vi "Proyecto finall.vi"() -> ()   [LabVIEW 2023]
uses:
  <vilib>/userDefined/High Color/IMAQdx.ctl
  <vilib>/DAQmx/write.llb/DAQmx Write (Digital 1D Bool NChan 1Samp 1Line).vi
  <vilib>/addons/database/Connection.llb/DB Tools Open Connec (Path).vi
  <vilib>/addons/database/Connection.llb/Conn Execute.vi
  <vilib>/addons/database/Recordset.llb/Rec Fetch Recordset Data (R).vi
  <vilib>/addons/database/Recordset.llb/Rec Destroy - Connection.vi
  <vilib>/DAQmx/miscellaneous.llb/DAQmx Fill In Error Info.vi
  <vilib>/addons/database/NI_Database_API.lvlib
  <vilib>/vision/driver/NI_Vision_Acquisition_Software.lvlib
panel:
  out "crujos 2":u16(ring)=1
  out "doros 2":u16(ring)=1
  out "cheetines 2":u16(ring)=1
  out "Gansito 2":u16(ring)=1
  out "Chips 2":u16(ring)=1
  out "Takis 2":u16(ring)=1
  out "SALDO":i32
  in  "Stop Button":bool
  out "Total Carrito":dbl=19.0
  in  "crujitos1":dbl min=0.0
  in  "doritos1":dbl min=0.0
  in  "chettos1":dbl min=0.0
  in  "chips1":dbl min=0.0
  in  "gansito1":dbl min=0.0
  in  "takis1":dbl min=0.0
  in  "STOP PROGRAMA":bool
  out "Takis":u16(ring)=1
  in  "disponibilidad tak":dbl=3.0 min=0.0 max=3.0
  in  "SaldoAux":dbl=100.0
  in  "Comprar":bool
  out "crujos":u16(ring)=3
  in  "disponibilidad cruji":dbl=3.0 min=0.0 max=3.0
  in  "crujitos":bool
  out "doros":u16(ring)=2
  in  "disponibilidad dori":dbl=3.0 min=0.0 max=3.0
  in  "doritos":bool
  out "cheetines":u16(ring)=2
  in  "disponibilidad chee":dbl=3.0 min=0.0 max=3.0
  in  "cheetos":bool
  out "String (OCR/OCV 1)":string="      "
  in  "File Path (OCR/OCV 1)":path=path "C:/Users/miagu/OneDrive/Escritorio/NUMBER.abc"
  out "Image":T1(plugin-control)
  out "Gansito":u16(ring)=2
  out "Chips":u16(ring)=2
  in  "disponibilidad gans":dbl=3.0 min=0.0 max=3.0
  in  "Disponibilidad chi":dbl=3.0 min=0.0 max=3.0
  in  "UDL":path=path "C:/Users/Dell/Desktop/maquina.udl"
  in  "gansito":bool
  in  "chips":bool
  in  "takis":bool
  out "Numeric 3":i32
  # "Carrito"
  # "Agregar Objetos"
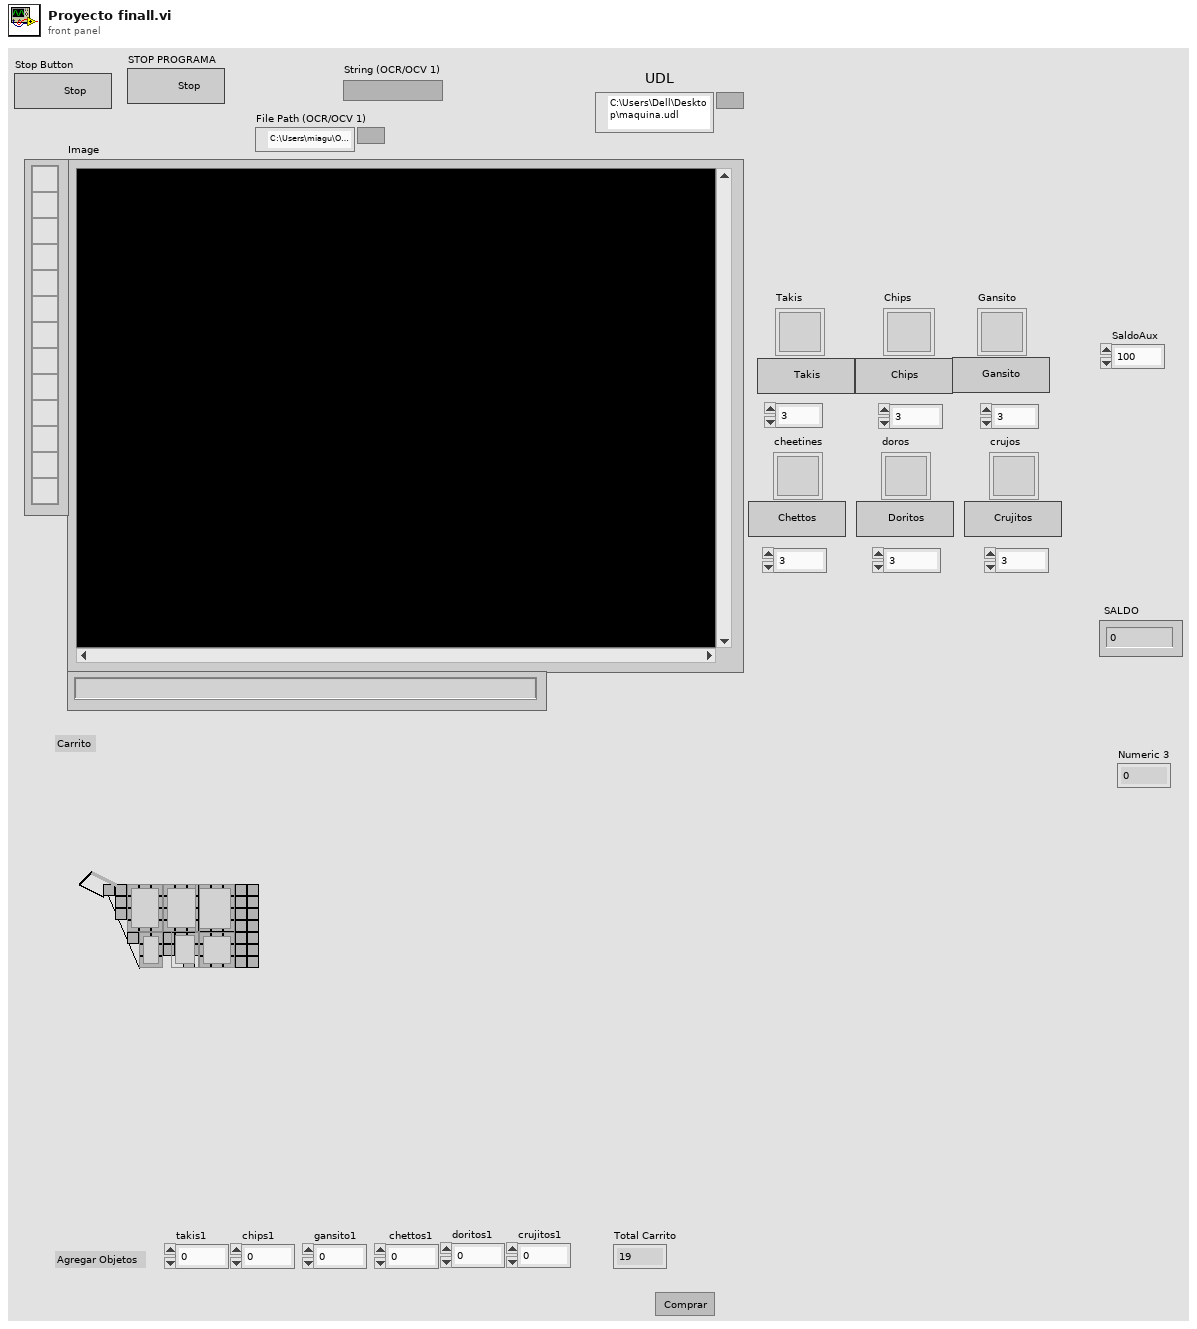
[diagram p1: front panel]
types:
  T1 = typedef "IMAQ Image.ctl" = refnum<image>
  T2 = cluster{"Threshold Data":cluster{"Method":enum16{"Fixed Range", "Uniform", "Linear", "Non Linear", "Local", "Color"}, "Looking for":u32, "Color Mode":u32, "Kernel Size":cluster{"Width":i32, "Height":i32}, "Ranges":cluster{"Min":i32, "Max":i32}[]}, "Reject Border":bool, "Number Of Erosions":i32, "Size & Spacing":cluster{"Segment Algorithm":u16, "Min Bounding Rect Width":i32, "Max Bounding Rect Width":i32, "Min Bounding Rect Height":i32, "Max Bounding Rect Height":i32, "Min Character Size":i32, "Max Character Size":i32, "Min Char Spacing":i32, "Max Horiz Element Spacing":i32, "Max Vert Element Spacing":i32, "Max Space Distance":i32}, "Read Options":cluster{"Read Strategy":i32, "Read Resolution":i32, "Scale Dependant":bool, "Aspect Ratio":i32, "Acceptance Level":i32, "Substitution Character":string, "MultiLine":bool}, "Valid Characters":cluster{"Pre-defined characters":i32, "User-defined characters":string}[], "Use Text Pattern":bool, "Orientation":u32, "# Lines Expected":u32, "Number of Blocks":i32}
  T3 = typedef "IMAQdx.ctl" = refnum<k21>
  T4 = cluster{"Global Rectangle":i32[], "Contours":cluster{"Contour Type":u32, "ROI Type":u32, "Points":i32[]}[]}
  T5 = typedef "NI_Database_API.lvlib/Conn ObjectReference.ctl" = refnum<k1>
  T6 = typedef "NI_Database_API.lvlib/Rec ObjectReference.ctl" = refnum<k1>
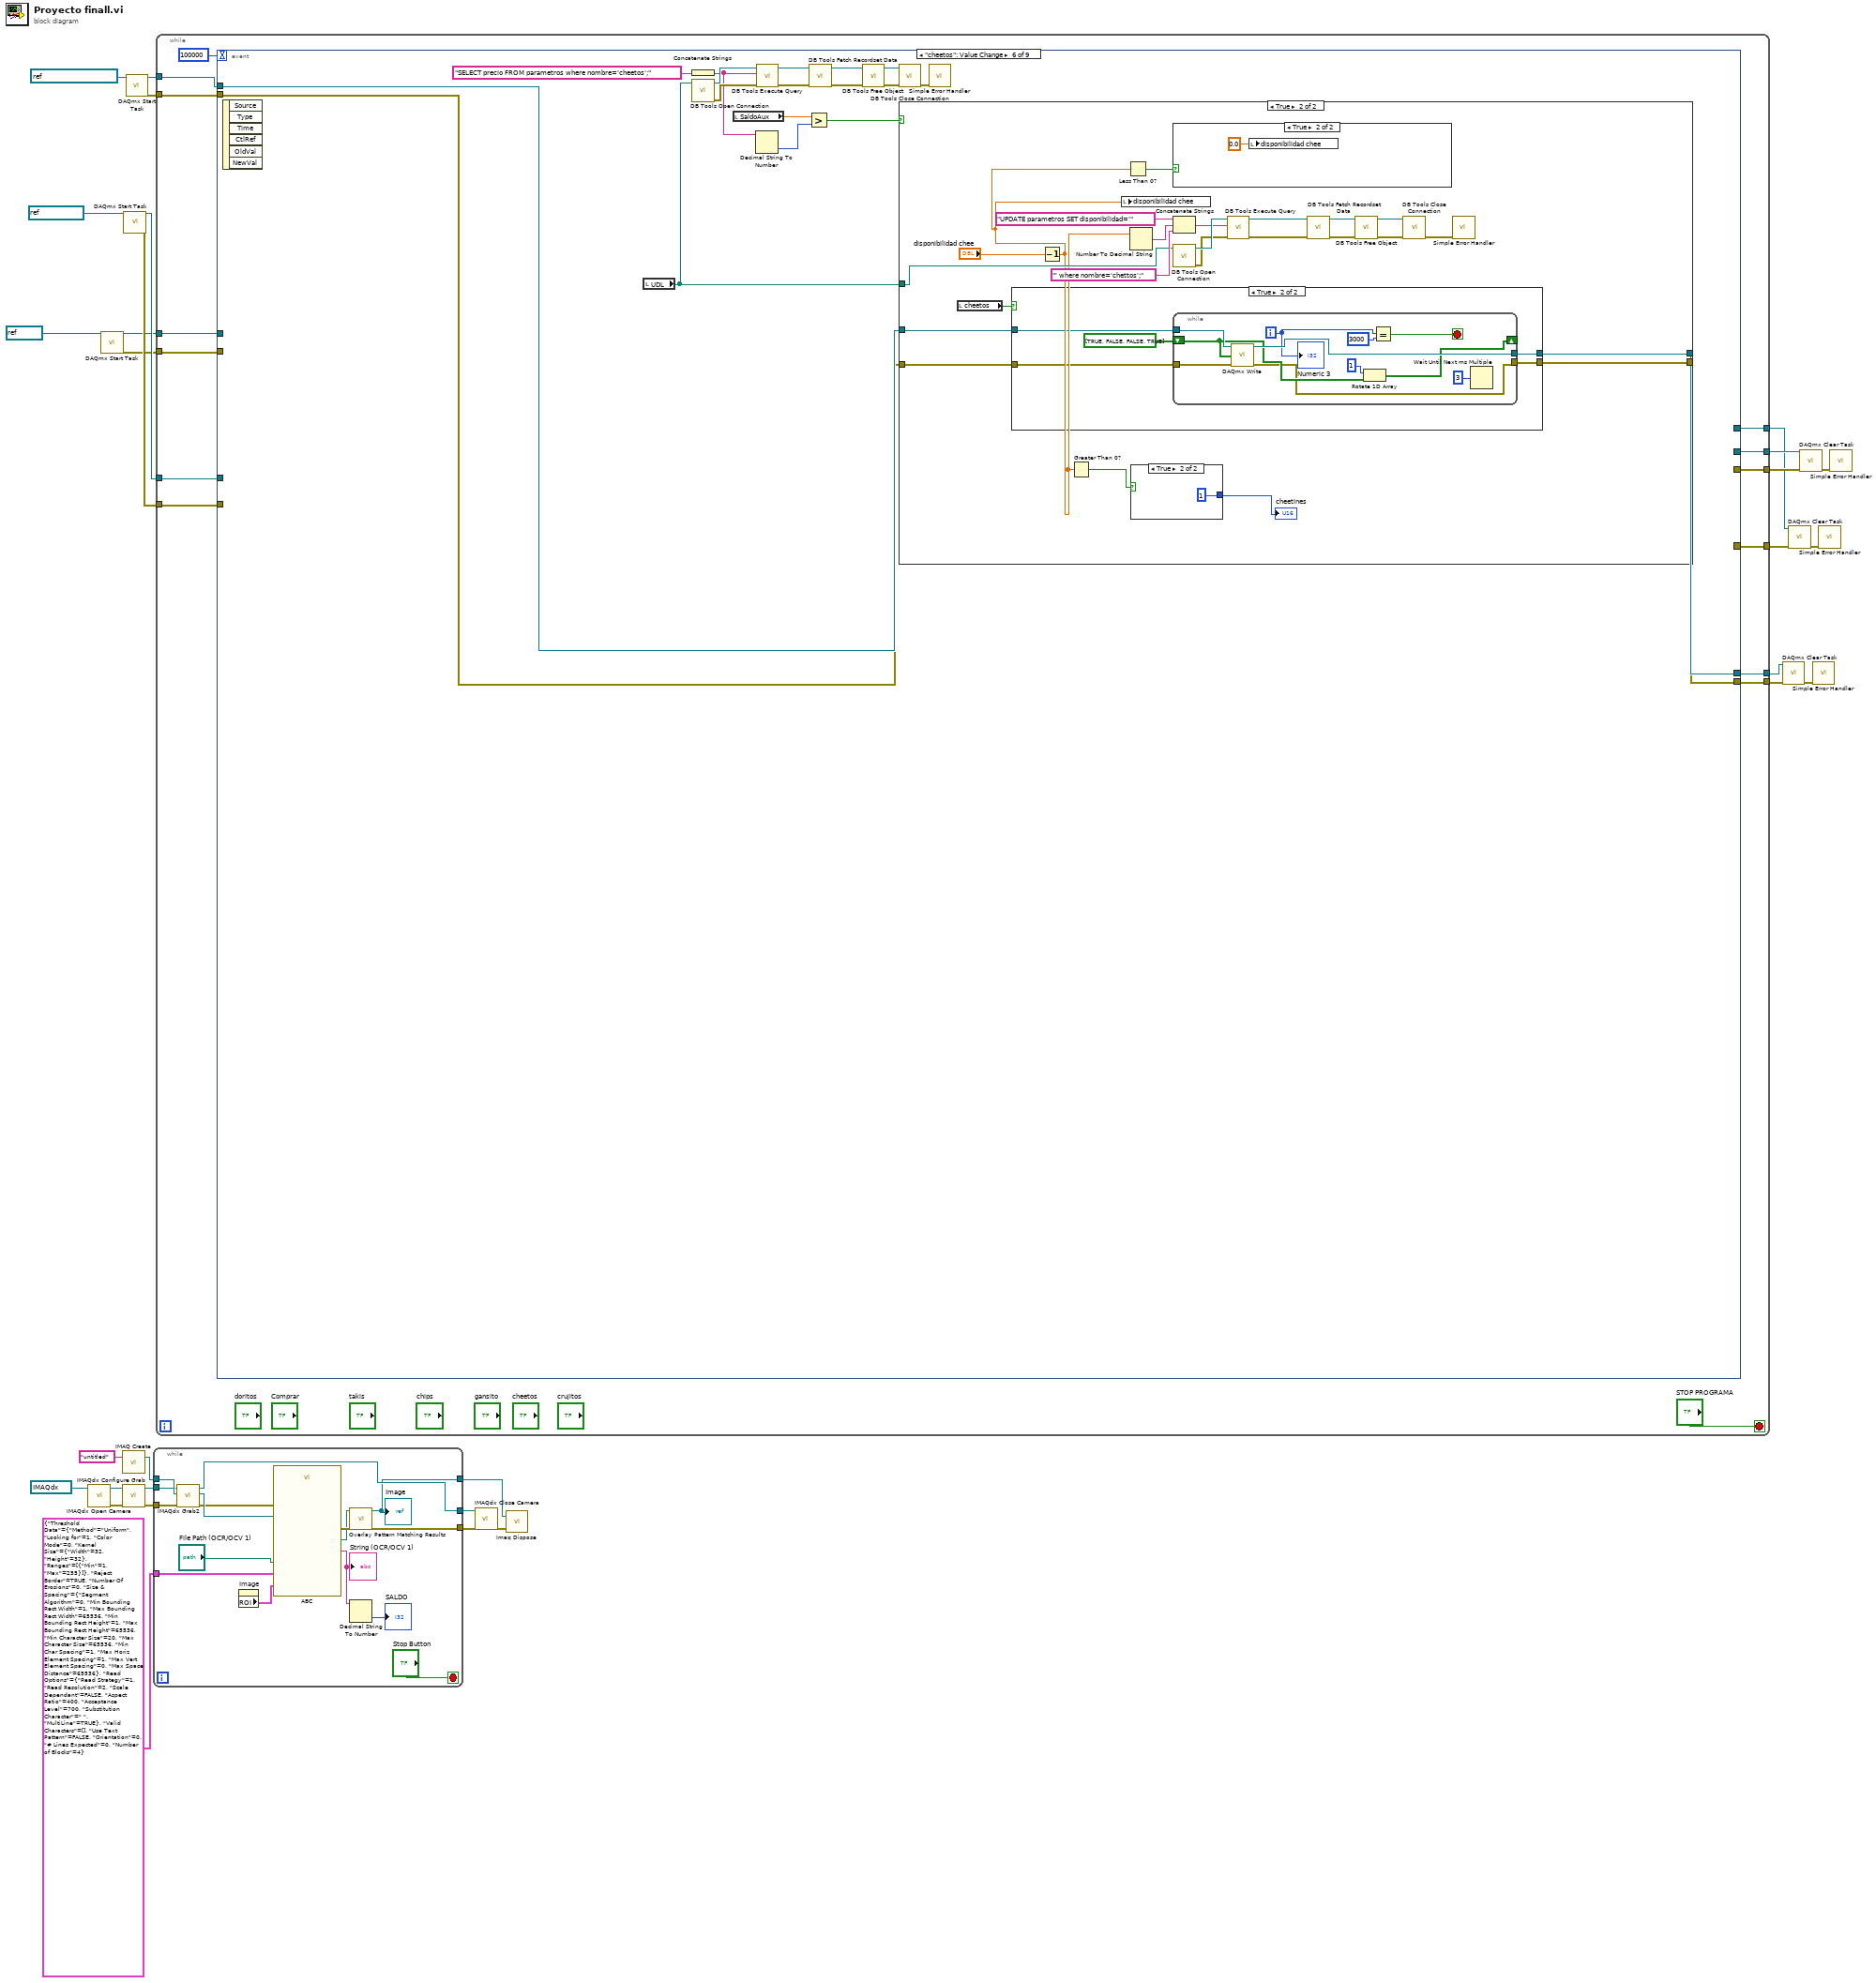
[diagram p0: block diagram]
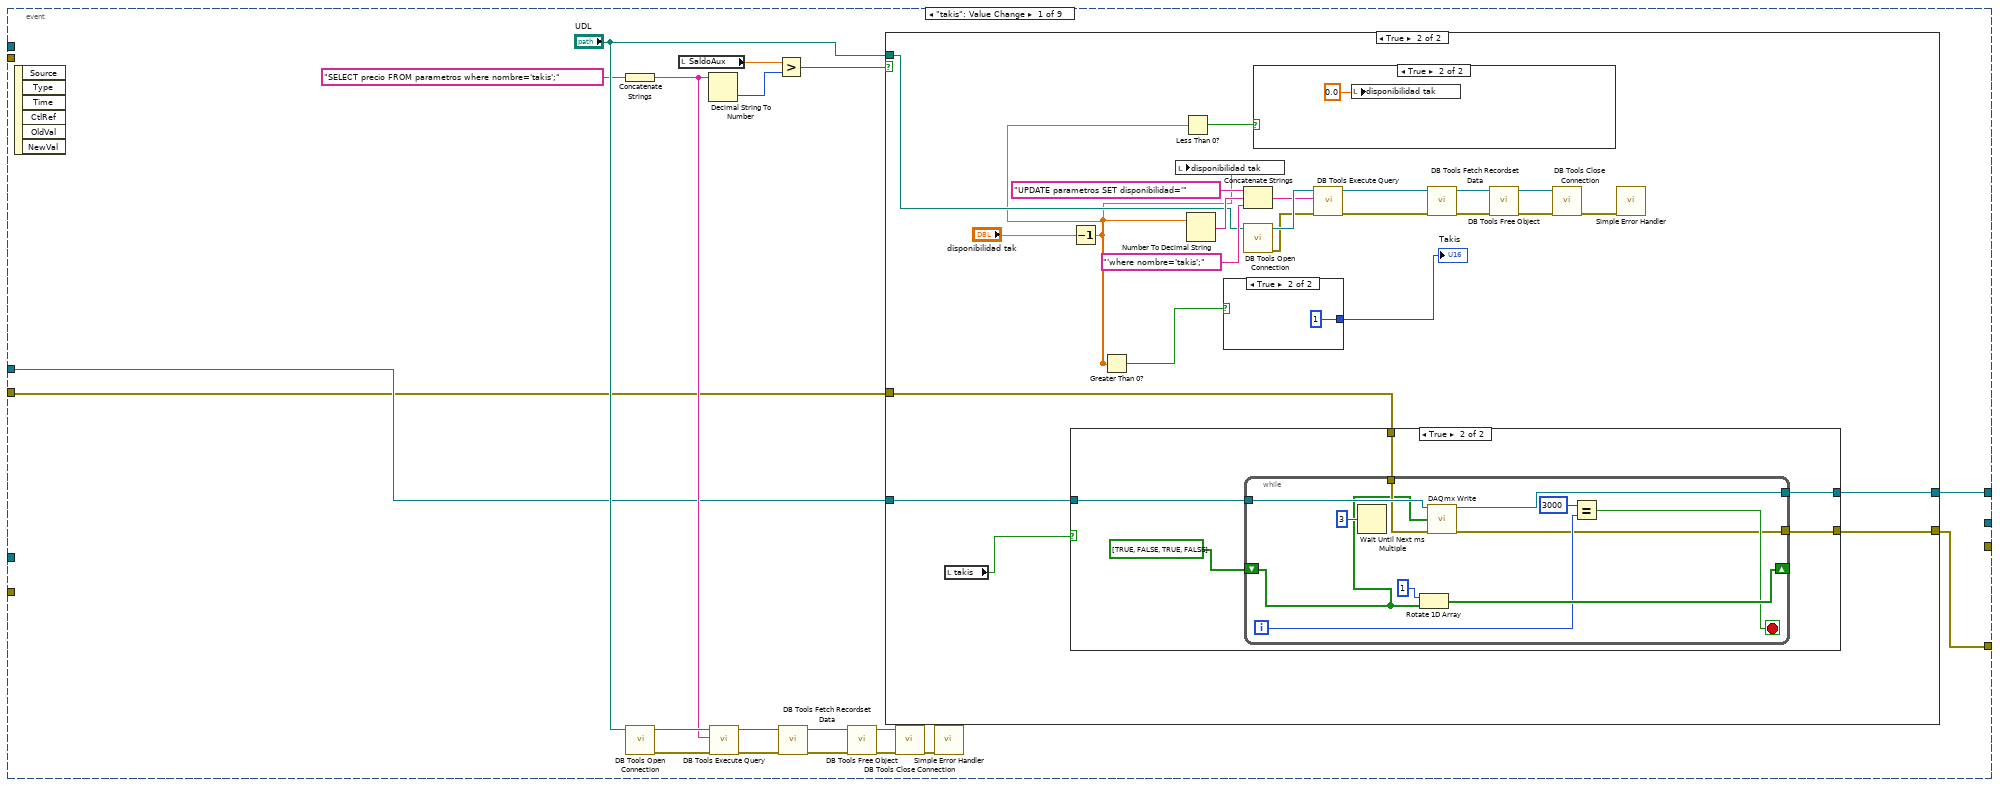
[diagram p2: hidden frame]
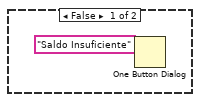
[diagram p3: hidden frame]
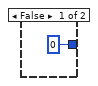
[diagram p5: hidden frame]
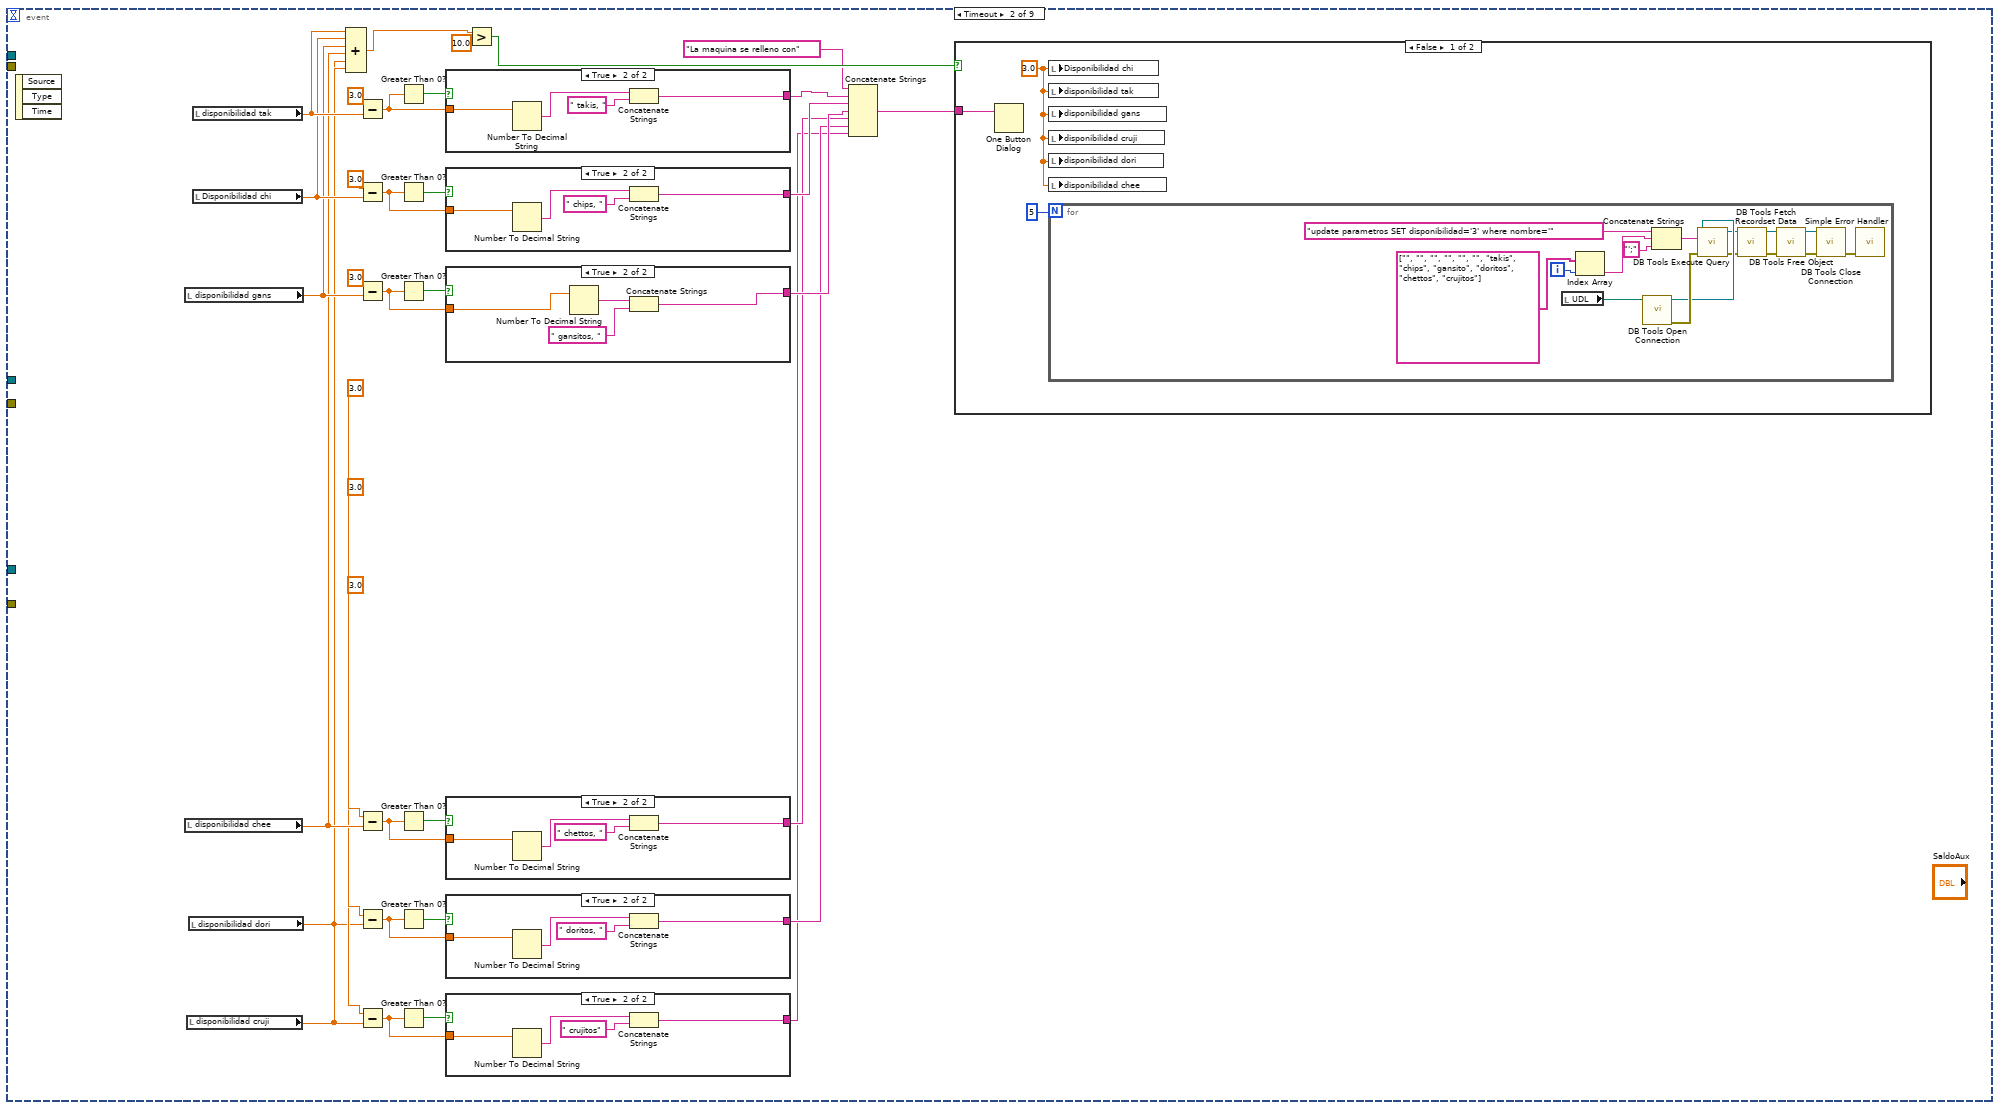
[diagram p7: hidden frame]
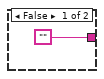
[diagram p8: hidden frame]
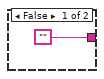
[diagram p9: hidden frame]
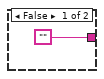
[diagram p10: hidden frame]
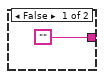
[diagram p11: hidden frame]
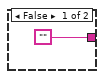
[diagram p12: hidden frame]
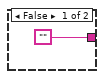
[diagram p13: hidden frame]
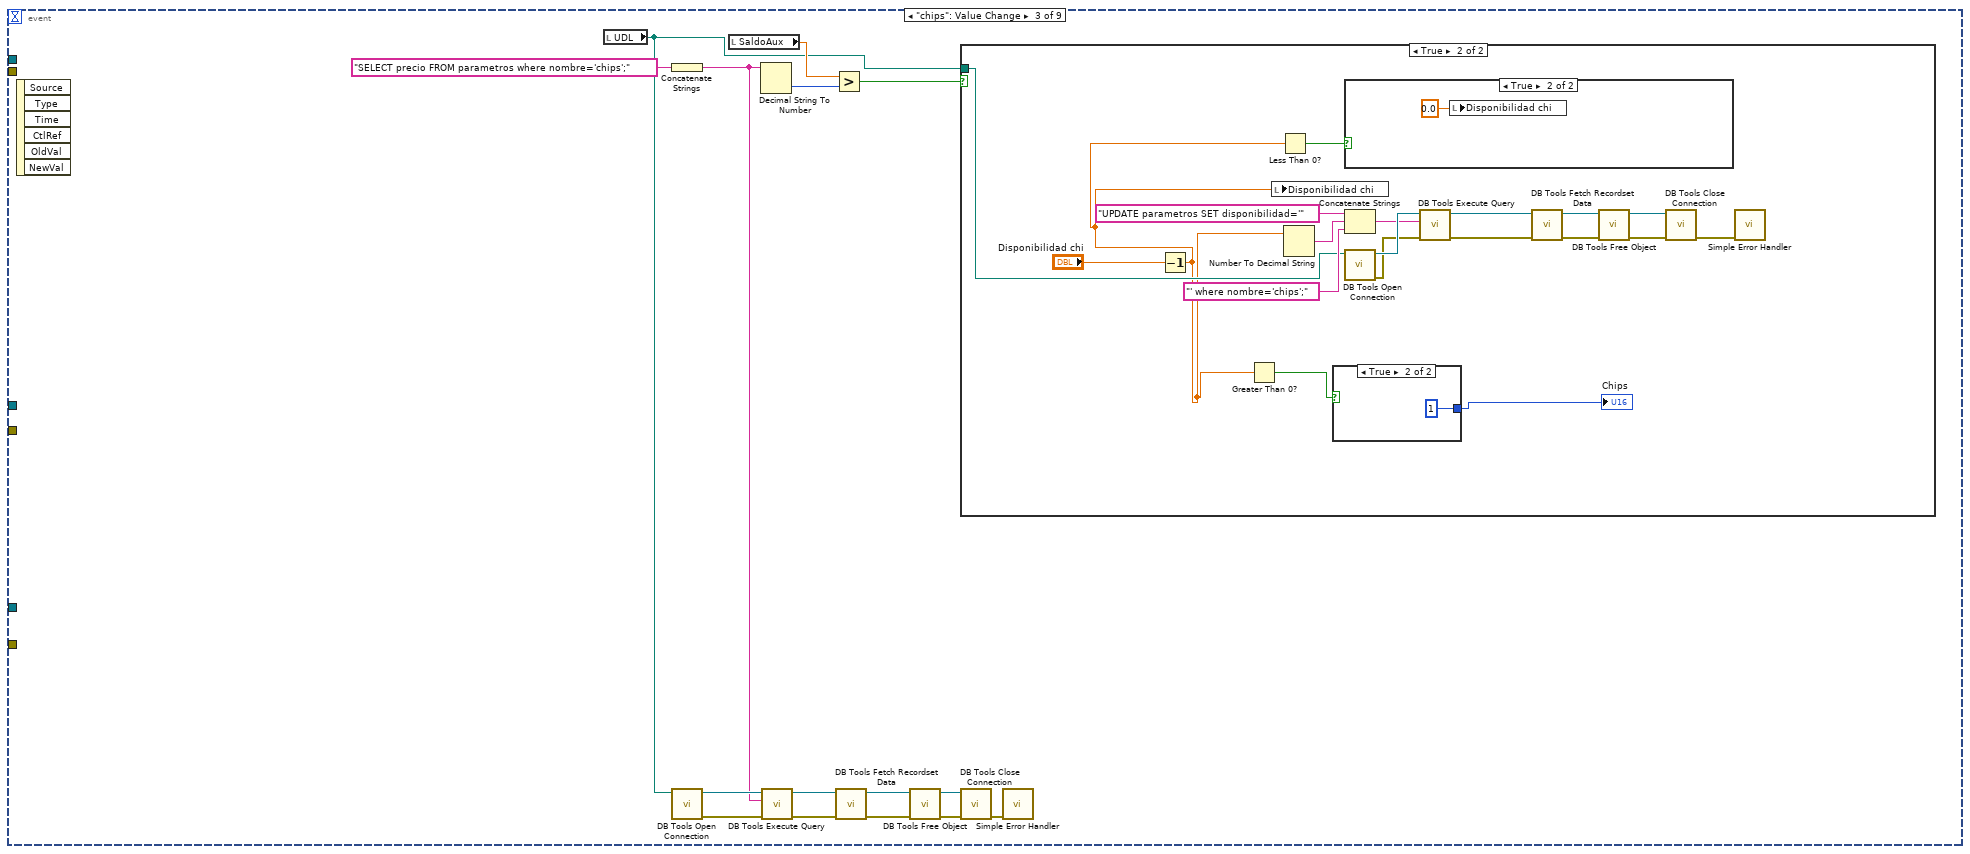
[diagram p15: hidden frame]
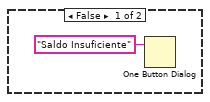
[diagram p16: hidden frame]
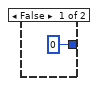
[diagram p17: hidden frame]
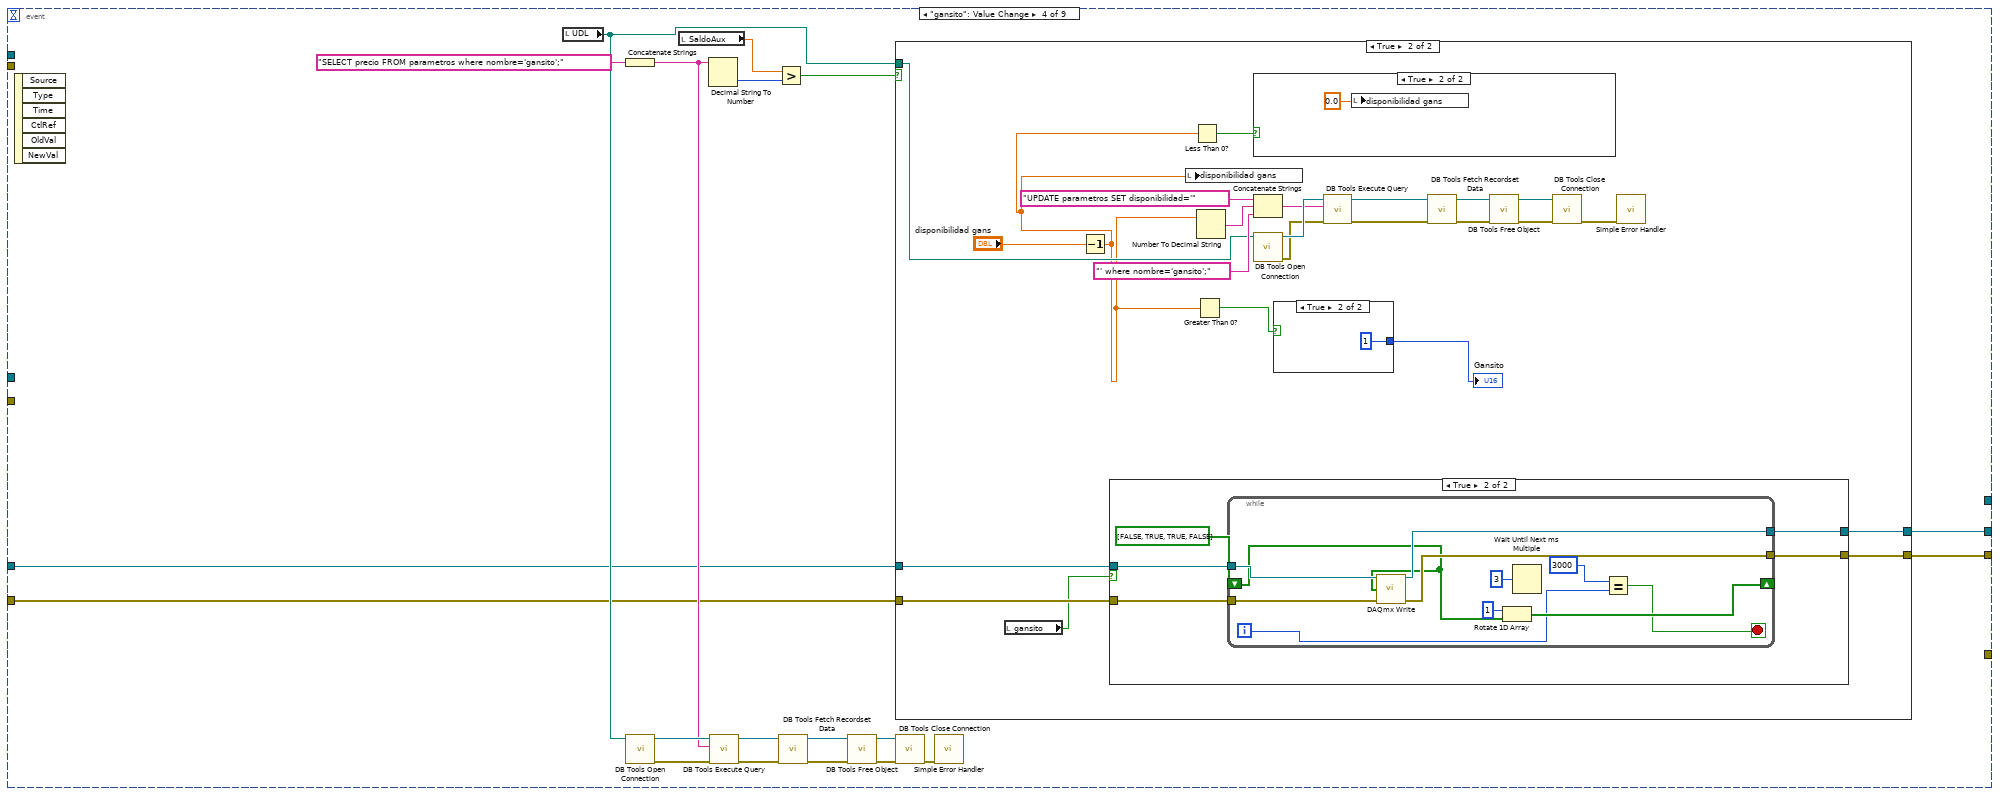
[diagram p19: hidden frame]
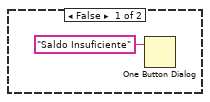
[diagram p20: hidden frame]
diagram:
  n1 = call <vilib>:"IMAQdx Open Camera.vi"("Session In"=T3 "cam1") -> ("error out"=w28:errorcluster, "Session Out"=w29:T3)  [unwired: 9 in]
  n2 = call <vilib>:"DAQmx Start Task.vi"("task/channels in"=refnum<k21> "out3") -> ("task out"=w5:refnum<k21>, "error out"=w4:errorcluster)  [unwired: 13 in]
  n3 = call "IMAQ Create"("Image Name"="untitled") -> ("New Image"=w18:T1)  [unwired: 4 in, 1 out]
  n4 = call <vilib>:"IMAQdx Configure Grab.vi"("error in"=w28, "Session In"=w29) -> ("error out"=w19:errorcluster, "Session Out"=w17:T3)  [unwired: 8 in]
  n5 = call <vilib>:"DAQmx Start Task.vi"("task/channels in"=refnum<k21> "OutTask2") -> ("task out"=w8:refnum<k21>, "error out"=w7:errorcluster)  [unwired: 13 in]
  n6 = call <vilib>:"DAQmx Start Task.vi"("task/channels in"=refnum<k21> "MyDigitalOutTask") -> ("task out"=w21:refnum<k21>, "error out"=w20:errorcluster)  [unwired: 13 in]
  n7 = while {
    tunnel: w19 -> [w45]
    tunnel: w18 -> [w44]
    tunnel: w17 -> [w43]
    tunnel: [w42] -> w16
    tunnel: T2 {"Threshold Data"={"Method"=enum."Uniform", "Looking for"=1, "Color Mode"=0, "Kernel Size"={"Width"=32, "Height"=32}, "Ranges"=[{"Min"=1, "Max"=255}]}, "Reject Border"=TRUE, "Number Of Erosions"=0, "Size & Spacing"={"Segment Algorithm"=0, "Min Bounding Rect Width"=1, "Max Bounding Rect Width"=65536, "Min Bounding Rect Height"=1, "Max Bounding Rect Height"=65536, "Min Character Size"=20, "Max Character Size"=65536, "Min Char Spacing"=1, "Max Horiz Element Spacing"=1, "Max Vert Element Spacing"=0, "Max Space Distance"=65536}, "Read Options"={"Read Strategy"=1, "Read Resolution"=2, "Scale Dependant"=FALSE, "Aspect Ratio"=400, "Acceptance Level"=700, "Substitution Character"=" ", "MultiLine"=TRUE}, "Valid Characters"=[], "Use Text Pattern"=FALSE, "Orientation"=0, "# Lines Expected"=0, "Number of Blocks"=4} ("Parameters (OCR/OCV 1)") -> [w38]
    tunnel: [w32] -> w14
    tunnel: [w31] -> w13
    stop <- "Stop Button" stop-if-true
    n8 = call <vilib>:"IMAQdx Grab2.vi"("error in"=w45, "Image In"=w44, "Session In"=w43) -> ("error out"=w37:errorcluster, "Image Out"=w41:T1, "Session Out"=w42:T3)  [unwired: 5 in, 1 out]
    n9 = property on="Image" class="ImageControl"() -> ("ROI"=w40:T4)  [unwired: 2 in, 2 out]
    n10 = call "ABC.vi"("Image In"=w41, "ROI Descriptor (OCR/OCV 1)"=w40, "File Path (OCR/OCV 1)"="File Path (OCR/OCV 1)", "Parameters (OCR/OCV 1)"=w38, "error in"=w37) -> ("Image Out"=w33:T1, "String (OCR/OCV 1)"=w35:string, "error out"=w34:errorcluster)  [unwired: 20 in]
    "String (OCR/OCV 1)" <- w35
    n11 = call "Overlay Pattern Matching Results.vi"("error in"=w34, "Image"=w33) -> ("error out"=w32:errorcluster, "Image Out"=w31:T1)  [unwired: 8 in]
    "Image" <- w31
    n12 = Decimal String To Number(string=w35) -> (number=→"SALDO":i32)  [unwired: 2 in, 1 out]
  }
  n13 = while {
    tunnel: [w59] -> w24
    tunnel: [w58] -> w23
    tunnel: w21 -> [w57]
    tunnel: w20 -> [w56]
    tunnel: [w54] -> w11
    tunnel: [w53] -> w9
    tunnel: w8 -> [w52]
    tunnel: w7 -> [w51]
    tunnel: w5 -> [w50]
    tunnel: w4 -> [w49]
    tunnel: [w48] -> w2
    tunnel: [w47] -> w1
    stop <- "STOP PROGRAMA" stop-if-true
    n14 = event shown="[5] \"cheetos\": Value Change" {
      selector: _ -> [_ _ _ _ _ _ _ _ _]
      dyn-events: _ -> [_ _ _ _ _ _ _ _ _]
      timeout: 100000 -> [_ _ _ _ _ _ _ _ _]
      tunnel: [_ _ _ _ _ w459 _ _ _] -> w59
      tunnel: [_ _ _ _ _ w458 _ _ _] -> w58
      tunnel: w57 -> [_ _ _ _ _ w457 _ _ _]
      tunnel: w56 -> [_ _ _ _ _ w456 _ _ _]
      tunnel: [_ _ _ w249 _ _ _ _ _] -> w54
      tunnel: [_ _ _ w248 _ _ _ _ _] -> w53
      tunnel: w52 -> [_ _ _ w247 _ _ _ _ _]
      tunnel: w51 -> [_ _ _ w246 _ _ _ _ _]
      tunnel: w50 -> [w64 _ _ _ _ _ _ _ _]
      tunnel: w49 -> [w63 _ _ _ _ _ _ _ _]
      tunnel: [w62 _ _ _ _ _ _ _ _] -> w48
      tunnel: [w61 _ _ _ _ _ _ _ _] -> w47
      event "takis": Value Change {
        n15 = event-data() -> ()  [unwired: 1 in, 6 out]
        n16 = Concatenate Strings("SELECT precio FROM parametros where nombre='takis';") -> (w65:string)
        n17 = call-poly <vilib>:"DB Tools Open Connection.vi"("connection information"="UDL") -> ("error out"=w75:errorcluster, "connection reference"=w74:T5)  [unwired: 7 in]
        n18 = local read "SaldoAux"() -> (w69:dbl)
        n19 = Decimal String To Number(string=w65) -> (number=w70:i32)  [unwired: 2 in, 1 out]
        n20 = call-poly <vilib>:"DB Tools Execute Query.vi"("error in (no error)"=w75, "SQL query"=w65, "connection reference"=w74) -> ("error out"=w79:errorcluster, "recordset reference"=w73:T6)  [unwired: 5 in]
        n21 = Greater?(x=w69, y=w70) -> (0:w68:bool)
        n22 = call-poly <vilib>:"DB Tools Fetch Recordset Data.vi"("error in (no error)"=w79, "recordset reference"=w73) -> ("error out"=w76:errorcluster, "recordset reference out"=w72:T6)  [unwired: 3 in, 1 out]
        n23 = call-poly <vilib>:"DB Tools Free Object.vi"("error in (no error)"=w76, "recordset reference"=w72) -> ("error out"=w77:errorcluster, "connection reference"=w71:T5)  [unwired: 8 in]
        n24 = case shown="True" w68 {
          tunnel: "UDL" -> [_ w89]
          tunnel: w64 -> [_ w85]
          tunnel: w63 -> [_ w84]
          tunnel: [_ w83] -> w62
          tunnel: [_ w82] -> w61
          frame False {
            n25 = One Button Dialog(message="Saldo Insuficiente") -> ()  [unwired: 1 in, 1 out]
          }
          frame True {
            n26 = local read "takis"() -> (w81:bool)
            n27 = case shown="True" w81 {
              tunnel: w85 -> [_ w109]
              tunnel: w84 -> [_ w108]
              tunnel: [_ w106] -> w83
              tunnel: [_ w105] -> w82
              frame False {
              }
              frame True {
                n28 = while {
                  shift-right: [w115] -> _
                  shift-left: bool[] [TRUE, FALSE, TRUE, FALSE] -> [w114]
                  tunnel: w109 -> [w117]
                  tunnel: w108 -> [w116]
                  tunnel: [w111] -> w106
                  tunnel: [w110] -> w105
                  i -> [w113]
                  stop <- w112 stop-if-true
                  n29 = Wait Until Next ms Multiple(millisecond multiple=u32 3) -> ()  [unwired: 1 out]
                  n30 = Rotate 1D Array(1:w114, 2:1 ("n")) -> (0:w115:bool[])
                  n31 = call-poly <vilib>:"DAQmx Write.vi"("task/channels in"=w117, "data"=w114, "error in"=w116) -> ("task out"=w111:refnum<k21>, "error out"=w110:errorcluster)  [unwired: 10 in, 1 out]
                  n32 = Equal?(x=3000, y=w113) -> (x = y?=w112:bool)
                }
              }
            }
            n33 = Decrement(x="disponibilidad tak") -> (x-1=w86:dbl)
            n34 = Greater Than 0?(x=w86) -> (x > 0?=w88:bool)
            n35 = local write "disponibilidad tak"(w86) -> ()
            n36 = Less Than 0?(x=w86) -> (x < 0?=w92:bool)
            n37 = Number To Decimal String(number=w86) -> (decimal integer string=w91:string)  [unwired: 1 in]
            n38 = case shown="True" w88 {
              tunnel: [u16 0 ("crujos") u16 1 ("crujos")] -> w87
              frame False {
              }
              frame True {
              }
            }
            "Takis" <- w87
            n39 = Concatenate Strings("UPDATE parametros SET disponibilidad='", w91, "'where nombre='takis';" ("string")) -> (w93:string)
            n40 = call-poly <vilib>:"DB Tools Open Connection.vi"("connection information"=w89) -> ("error out"=w96:errorcluster, "connection reference"=w102:T5)  [unwired: 7 in]
            n41 = case shown="True" w92 {
              frame False {
              }
              frame True {
                n42 = local write "disponibilidad tak"(0.0 ("TAKIS")) -> ()
              }
            }
            n43 = call-poly <vilib>:"DB Tools Execute Query.vi"("error in (no error)"=w96, "SQL query"=w93, "connection reference"=w102) -> ("error out"=w104:errorcluster, "recordset reference"=w103:T6)  [unwired: 5 in]
            n44 = call-poly <vilib>:"DB Tools Fetch Recordset Data.vi"("error in (no error)"=w104, "recordset reference"=w103) -> ("error out"=w97:errorcluster, "recordset reference out"=w101:T6)  [unwired: 3 in, 1 out]
            n45 = call-poly <vilib>:"DB Tools Free Object.vi"("error in (no error)"=w97, "recordset reference"=w101) -> ("error out"=w98:errorcluster, "connection reference"=w100:T5)  [unwired: 8 in]
            n46 = call <vilib>:"DB Tools Close Connection.vi"("error in (no error)"=w98, "connection reference"=w100) -> ("error out"=w99:errorcluster)  [unwired: 5 in]
            n47 = call <vilib>:"Simple Error Handler.vi"("error in (no error)"=w99) -> ()  [unwired: 4 in, 5 out]
          }
        }
        n48 = call <vilib>:"DB Tools Close Connection.vi"("error in (no error)"=w77, "connection reference"=w71) -> ("error out"=w78:errorcluster)  [unwired: 5 in]
        n49 = call <vilib>:"Simple Error Handler.vi"("error in (no error)"=w78) -> ()  [unwired: 4 in, 5 out]
      }
      event Timeout {
        n50 = event-data() -> ()  [unwired: 1 in, 3 out]
        n51 = local read "disponibilidad gans"() -> (w140:dbl)
        n52 = local read "disponibilidad chee"() -> (w136:dbl)
        n53 = local read "disponibilidad cruji"() -> (w125:dbl)
        n54 = local read "disponibilidad dori"() -> (w126:dbl)
        n55 = local read "disponibilidad tak"() -> (w155:dbl)
        n56 = local read "Disponibilidad chi"() -> (w148:dbl)
        n57 = Compound Arithmetic op=ADD(w155, w148, w140, w136, w125, w126) -> (w158:dbl)
        n58 = Subtract(x=3.0, y=w155) -> (x-y=w151:dbl)
        n59 = Subtract(x=3.0, y=w148) -> (x-y=w149:dbl)
        n60 = Subtract(x=3.0, y=w140) -> (x-y=w144:dbl)
        n61 = Subtract(x=3.0, y=w136) -> (x-y=w138:dbl)
        n62 = Subtract(x=3.0, y=w126) -> (x-y=w133:dbl)
        n63 = Subtract(x=3.0, y=w125) -> (x-y=w129:dbl)
        n64 = Greater Than 0?(x=w151) -> (x > 0?=w153:bool)
        n65 = Greater Than 0?(x=w149) -> (x > 0?=w143:bool)
        n66 = Greater Than 0?(x=w144) -> (x > 0?=w142:bool)
        n67 = Greater Than 0?(x=w138) -> (x > 0?=w137:bool)
        n68 = Greater Than 0?(x=w133) -> (x > 0?=w132:bool)
        n69 = Greater Than 0?(x=w129) -> (x > 0?=w128:bool)
        n70 = case shown="True" w153 {
          tunnel: w151 -> [_ w188]
          tunnel: ["" w185] -> w147
          frame False {
          }
          frame True {
            n71 = Number To Decimal String(number=w188) -> (decimal integer string=w187:string)  [unwired: 1 in]
            n72 = Concatenate Strings(w187, " takis, " ("string")) -> (w185:string)
          }
        }
        n73 = case shown="True" w143 {
          tunnel: w149 -> [_ w183]
          tunnel: ["" w180] -> w146
          frame False {
          }
          frame True {
            n74 = Number To Decimal String(number=w183) -> (decimal integer string=w182:string)  [unwired: 1 in]
            n75 = Concatenate Strings(w182, " chips, " ("string")) -> (w180:string)
          }
        }
        n76 = case shown="True" w142 {
          tunnel: w144 -> [_ w178]
          tunnel: ["" w175] -> w141
          frame False {
          }
          frame True {
            n77 = Number To Decimal String(number=w178) -> (decimal integer string=w177:string)  [unwired: 1 in]
            n78 = Concatenate Strings(w177, " gansitos, " ("string")) -> (w175:string)
          }
        }
        n79 = case shown="True" w137 {
          tunnel: w138 -> [_ w173]
          tunnel: ["" w170] -> w135
          frame False {
          }
          frame True {
            n80 = Number To Decimal String(number=w173) -> (decimal integer string=w172:string)  [unwired: 1 in]
            n81 = Concatenate Strings(w172, " chettos, " ("string")) -> (w170:string)
          }
        }
        n82 = case shown="True" w132 {
          tunnel: w133 -> [_ w168]
          tunnel: ["" w165] -> w131
          frame False {
          }
          frame True {
            n83 = Number To Decimal String(number=w168) -> (decimal integer string=w167:string)  [unwired: 1 in]
            n84 = Concatenate Strings(w167, " doritos, " ("string")) -> (w165:string)
          }
        }
        n85 = case shown="True" w128 {
          tunnel: w129 -> [_ w163]
          tunnel: ["" w160] -> w127
          frame False {
          }
          frame True {
            n86 = Number To Decimal String(number=w163) -> (decimal integer string=w162:string)  [unwired: 1 in]
            n87 = Concatenate Strings(w162, " crujitos" ("string")) -> (w160:string)
          }
        }
        n88 = Greater?(x=w158, y=10.0) -> (0:w157:bool)
        n89 = Concatenate Strings("La maquina se relleno con" ("string"), w147, w146, w141, w135, w131, w127) -> (w124:string)
        n90 = case shown="False" w157 {
          tunnel: w124 -> [w189 _]
          frame False {
            w190 = 3.0
            n91 = One Button Dialog(message=w189) -> ()  [unwired: 1 in, 1 out]
            n92 = local write "Disponibilidad chi"(w190) -> ()
            n93 = local write "disponibilidad tak"(w190) -> ()
            n94 = local write "disponibilidad gans"(w190) -> ()
            n95 = local write "disponibilidad cruji"(w190) -> ()
            n96 = local write "disponibilidad dori"(w190) -> ()
            n97 = local write "disponibilidad chee"(w190) -> ()
            n98 = for {
              N: 5 -> [_]
              i -> [w196]
              n99 = local read "UDL"() -> (w207:path)
              n100 = Index Array(array=string[] ["", "", "", "", "", "", "takis", "chips", "gansito", "doritos", "chettos", "crujitos"], index=w196) -> (element=w194:string)
              n101 = call-poly <vilib>:"DB Tools Open Connection.vi"("connection information"=w207) -> ("error out"=w206:errorcluster, "connection reference"=w200:T5)  [unwired: 7 in]
              n102 = Concatenate Strings("update parametros SET disponibilidad='3' where nombre='" ("string"), w194, "';" ("string")) -> (w192:string)
              n103 = call-poly <vilib>:"DB Tools Execute Query.vi"("error in (no error)"=w206, "SQL query"=w192, "connection reference"=w200) -> ("error out"=w198:errorcluster, "recordset reference"=w199:T6)  [unwired: 5 in]
              n104 = call-poly <vilib>:"DB Tools Fetch Recordset Data.vi"("error in (no error)"=w198, "recordset reference"=w199) -> ("error out"=w205:errorcluster, "recordset reference out"=w201:T6)  [unwired: 3 in, 1 out]
              n105 = call-poly <vilib>:"DB Tools Free Object.vi"("error in (no error)"=w205, "recordset reference"=w201) -> ("error out"=w204:errorcluster, "connection reference"=w202:T5)  [unwired: 8 in]
              n106 = call <vilib>:"DB Tools Close Connection.vi"("error in (no error)"=w204, "connection reference"=w202) -> ("error out"=w203:errorcluster)  [unwired: 5 in]
              n107 = call <vilib>:"Simple Error Handler.vi"("error in (no error)"=w203) -> ()  [unwired: 4 in, 5 out]
            }
          }
          frame True {
          }
        }
      }
      event "chips": Value Change {
        n108 = event-data() -> ()  [unwired: 1 in, 6 out]
        n109 = local read "UDL"() -> (w211:path)
        n110 = Concatenate Strings("SELECT precio FROM parametros where nombre='chips';") -> (w208:string)
        n111 = call-poly <vilib>:"DB Tools Open Connection.vi"("connection information"=w211) -> ("error out"=w218:errorcluster, "connection reference"=w217:T5)  [unwired: 7 in]
        n112 = local read "SaldoAux"() -> (w212:dbl)
        n113 = Decimal String To Number(string=w208) -> (number=w213:i32)  [unwired: 2 in, 1 out]
        n114 = call-poly <vilib>:"DB Tools Execute Query.vi"("error in (no error)"=w218, "SQL query"=w208, "connection reference"=w217) -> ("error out"=w222:errorcluster, "recordset reference"=w216:T6)  [unwired: 5 in]
        n115 = Greater?(x=w212, y=w213) -> (0:w210:bool)
        n116 = call-poly <vilib>:"DB Tools Fetch Recordset Data.vi"("error in (no error)"=w222, "recordset reference"=w216) -> ("error out"=w219:errorcluster, "recordset reference out"=w215:T6)  [unwired: 3 in, 1 out]
        n117 = call-poly <vilib>:"DB Tools Free Object.vi"("error in (no error)"=w219, "recordset reference"=w215) -> ("error out"=w220:errorcluster, "connection reference"=w214:T5)  [unwired: 8 in]
        n118 = case shown="True" w210 {
          tunnel: w211 -> [_ w227]
          frame False {
            n119 = One Button Dialog(message="Saldo Insuficiente") -> ()  [unwired: 1 in, 1 out]
          }
          frame True {
            n120 = Decrement(x="Disponibilidad chi") -> (x-1=w224:dbl)
            n121 = Greater Than 0?(x=w224) -> (x > 0?=w226:bool)
            n122 = local write "Disponibilidad chi"(w224) -> ()
            n123 = Less Than 0?(x=w224) -> (x < 0?=w231:bool)
            n124 = Number To Decimal String(number=w224) -> (decimal integer string=w228:string)  [unwired: 1 in]
            n125 = case shown="True" w226 {
              tunnel: [u16 0 ("crujos") u16 1 ("crujos")] -> w225
              frame False {
              }
              frame True {
              }
            }
            "Chips" <- w225
            n126 = case shown="True" w231 {
              frame False {
              }
              frame True {
                n127 = local write "Disponibilidad chi"(0.0 ("TAKIS")) -> ()
              }
            }
            n128 = Concatenate Strings("UPDATE parametros SET disponibilidad='", w228, "' where nombre='chips';") -> (w230:string)
            n129 = call-poly <vilib>:"DB Tools Open Connection.vi"("connection information"=w227) -> ("error out"=w234:errorcluster, "connection reference"=w240:T5)  [unwired: 7 in]
            n130 = call-poly <vilib>:"DB Tools Execute Query.vi"("error in (no error)"=w234, "SQL query"=w230, "connection reference"=w240) -> ("error out"=w242:errorcluster, "recordset reference"=w241:T6)  [unwired: 5 in]
            n131 = call-poly <vilib>:"DB Tools Fetch Recordset Data.vi"("error in (no error)"=w242, "recordset reference"=w241) -> ("error out"=w235:errorcluster, "recordset reference out"=w239:T6)  [unwired: 3 in, 1 out]
            n132 = call-poly <vilib>:"DB Tools Free Object.vi"("error in (no error)"=w235, "recordset reference"=w239) -> ("error out"=w236:errorcluster, "connection reference"=w238:T5)  [unwired: 8 in]
            n133 = call <vilib>:"DB Tools Close Connection.vi"("error in (no error)"=w236, "connection reference"=w238) -> ("error out"=w237:errorcluster)  [unwired: 5 in]
            n134 = call <vilib>:"Simple Error Handler.vi"("error in (no error)"=w237) -> ()  [unwired: 4 in, 5 out]
          }
        }
        n135 = call <vilib>:"DB Tools Close Connection.vi"("error in (no error)"=w220, "connection reference"=w214) -> ("error out"=w221:errorcluster)  [unwired: 5 in]
        n136 = call <vilib>:"Simple Error Handler.vi"("error in (no error)"=w221) -> ()  [unwired: 4 in, 5 out]
      }
      event "gansito": Value Change {
        n137 = event-data() -> ()  [unwired: 1 in, 6 out]
        n138 = local read "UDL"() -> (w254:path)
        n139 = Concatenate Strings("SELECT precio FROM parametros where nombre='gansito';") -> (w250:string)
        n140 = call-poly <vilib>:"DB Tools Open Connection.vi"("connection information"=w254) -> ("error out"=w260:errorcluster, "connection reference"=w259:T5)  [unwired: 7 in]
        n141 = local read "SaldoAux"() -> (w252:dbl)
        n142 = Decimal String To Number(string=w250) -> (number=w255:i32)  [unwired: 2 in, 1 out]
        n143 = call-poly <vilib>:"DB Tools Execute Query.vi"("error in (no error)"=w260, "SQL query"=w250, "connection reference"=w259) -> ("error out"=w264:errorcluster, "recordset reference"=w258:T6)  [unwired: 5 in]
        n144 = Greater?(x=w252, y=w255) -> (0:w253:bool)
        n145 = call-poly <vilib>:"DB Tools Fetch Recordset Data.vi"("error in (no error)"=w264, "recordset reference"=w258) -> ("error out"=w261:errorcluster, "recordset reference out"=w257:T6)  [unwired: 3 in, 1 out]
        n146 = call-poly <vilib>:"DB Tools Free Object.vi"("error in (no error)"=w261, "recordset reference"=w257) -> ("error out"=w262:errorcluster, "connection reference"=w256:T5)  [unwired: 8 in]
        n147 = case shown="True" w253 {
          tunnel: w254 -> [_ w274]
          tunnel: [_ w270] -> w249
          tunnel: [_ w269] -> w248
          tunnel: w247 -> [_ w268]
          tunnel: w246 -> [_ w267]
          frame False {
            n148 = One Button Dialog(message="Saldo Insuficiente") -> ()  [unwired: 1 in, 1 out]
          }
          frame True {
            n149 = local read "gansito"() -> (w266:bool)
            n150 = Decrement(x="disponibilidad gans") -> (x-1=w271:dbl)
            n151 = case shown="True" w266 {
              tunnel: [_ w294] -> w270
              tunnel: [_ w293] -> w269
              tunnel: w268 -> [_ w292]
              tunnel: w267 -> [_ w291]
              frame False {
              }
              frame True {
                n152 = while {
                  tunnel: [w305] -> w294
                  tunnel: [w304] -> w293
                  tunnel: w292 -> [w303]
                  tunnel: w291 -> [w302]
                  shift-right: [w300] -> _
                  shift-left: bool[] [FALSE, TRUE, TRUE, FALSE] -> [w295]
                  i -> [w297]
                  stop <- w298 stop-if-true
                  n153 = call-poly <vilib>:"DAQmx Write.vi"("task/channels in"=w303, "data"=w295, "error in"=w302) -> ("task out"=w305:refnum<k21>, "error out"=w304:errorcluster)  [unwired: 10 in, 1 out]
                  n154 = Rotate 1D Array(1:w295, 2:1 ("n")) -> (0:w300:bool[])
                  n155 = Wait Until Next ms Multiple(millisecond multiple=u32 3) -> ()  [unwired: 1 out]
                  n156 = Equal?(x=3000, y=w297) -> (x = y?=w298:bool)
                }
              }
            }
            n157 = local write "disponibilidad gans"(w271) -> ()
            n158 = Less Than 0?(x=w271) -> (x < 0?=w277:bool)
            n159 = Greater Than 0?(x=w271) -> (x > 0?=w273:bool)
            n160 = Number To Decimal String(number=w271) -> (decimal integer string=w275:string)  [unwired: 1 in]
            n161 = case shown="True" w277 {
              frame False {
              }
              frame True {
                n162 = local write "disponibilidad gans"(0.0 ("TAKIS")) -> ()
              }
            }
            n163 = Concatenate Strings("UPDATE parametros SET disponibilidad='", w275, "' where nombre='gansito';") -> (w276:string)
            n164 = call-poly <vilib>:"DB Tools Open Connection.vi"("connection information"=w274) -> ("error out"=w281:errorcluster, "connection reference"=w287:T5)  [unwired: 7 in]
            n165 = case shown="True" w273 {
              tunnel: [u16 0 ("crujos") u16 1 ("crujos")] -> w272
              frame False {
              }
              frame True {
              }
            }
            "Gansito" <- w272
            n166 = call-poly <vilib>:"DB Tools Execute Query.vi"("error in (no error)"=w281, "SQL query"=w276, "connection reference"=w287) -> ("error out"=w289:errorcluster, "recordset reference"=w288:T6)  [unwired: 5 in]
            n167 = call-poly <vilib>:"DB Tools Fetch Recordset Data.vi"("error in (no error)"=w289, "recordset reference"=w288) -> ("error out"=w282:errorcluster, "recordset reference out"=w286:T6)  [unwired: 3 in, 1 out]
            n168 = call-poly <vilib>:"DB Tools Free Object.vi"("error in (no error)"=w282, "recordset reference"=w286) -> ("error out"=w283:errorcluster, "connection reference"=w285:T5)  [unwired: 8 in]
            n169 = call <vilib>:"DB Tools Close Connection.vi"("error in (no error)"=w283, "connection reference"=w285) -> ("error out"=w284:errorcluster)  [unwired: 5 in]
            n170 = call <vilib>:"Simple Error Handler.vi"("error in (no error)"=w284) -> ()  [unwired: 4 in, 5 out]
          }
        }
        n171 = call <vilib>:"DB Tools Close Connection.vi"("error in (no error)"=w262, "connection reference"=w256) -> ("error out"=w263:errorcluster)  [unwired: 5 in]
        n172 = call <vilib>:"Simple Error Handler.vi"("error in (no error)"=w263) -> ()  [unwired: 4 in, 5 out]
      }
      event "Comprar": Value Change {
        n173 = event-data() -> ()  [unwired: 1 in, 6 out]
        n174 = local read "Total Carrito"() -> (w309:dbl)
        n175 = local read "SaldoAux"() -> (w310:dbl)
        n176 = Greater Or Equal?(x=w310, y=w309) -> (x >= y?=w311:bool)
        n177 = case shown="True" w311 {
          frame False {
          }
          frame True {
            n178 = local read "Disponibilidad chi"() -> (w319:dbl)
            n179 = local read "disponibilidad tak"() -> (w321:dbl)
            n180 = local read "disponibilidad chee"() -> (w317:dbl)
            n181 = local read "disponibilidad gans"() -> (w318:dbl)
            n182 = local read "disponibilidad cruji"() -> (w313:dbl)
            n183 = local read "disponibilidad dori"() -> (w314:dbl)
            n184 = local read "chettos1"() -> (w327:dbl)
            n185 = local read "crujitos1"() -> (w324:dbl)
            n186 = local read "gansito1"() -> (w333:dbl)
            n187 = local read "doritos1"() -> (w325:dbl)
            n188 = local read "chips1"() -> (w334:dbl)
            n189 = local read "takis1"() -> (w345:dbl)
            n190 = Subtract(x=w313, y=w324) -> (x-y=w312:dbl)
            n191 = Subtract(x=w314, y=w325) -> (x-y=w315:dbl)
            n192 = Subtract(x=w317, y=w327) -> (x-y=w316:dbl)
            n193 = Subtract(x=w319, y=w334) -> (x-y=w320:dbl)
            n194 = Subtract(x=w321, y=w345) -> (x-y=w322:dbl)
            n195 = Subtract(x=w318, y=w333) -> (x-y=w332:dbl)
            n196 = local write "disponibilidad gans"(w332) -> ()
            n197 = Greater Or Equal?(x=w312, y=0.0 ("x")) -> (x >= y?=w335:bool)
            n198 = Greater Or Equal?(x=w315, y=0.0 ("x")) -> (x >= y?=w337:bool)
            n199 = Greater Or Equal?(x=w316, y=0.0 ("x")) -> (x >= y?=w339:bool)
            n200 = Greater Or Equal?(x=w332, y=0.0 ("x")) -> (x >= y?=w341:bool)
            n201 = Greater Or Equal?(x=w320, y=0.0 ("x")) -> (x >= y?=w343:bool)
            n202 = Greater Or Equal?(x=w322, y=0.0 ("x")) -> (x >= y?=w346:bool)
            n203 = case shown="False" w335 {
              tunnel: w312 -> [_ w407]
              tunnel: ["select nombre from parametros" w408] -> w323
              tunnel: w313 -> [w403 _]
              tunnel: w312 -> [_ w406]
              frame False {
                n204 = local write "disponibilidad cruji"(w403) -> ()
                n205 = One Button Dialog(message="Crujitos Insuficientes") -> ()  [unwired: 1 in, 1 out]
              }
              frame True {
                n206 = local write "disponibilidad cruji"(w406) -> ()
                n207 = Number To Decimal String(number=w407) -> (decimal integer string=w410:string)  [unwired: 1 in]
                n208 = Concatenate Strings("update parametros SET disponibilidad='", w410, " ' where nombre='crujitos';" ("string")) -> (w408:string)
              }
            }
            n209 = case shown="False" w337 {
              tunnel: w315 -> [_ w417]
              tunnel: ["select nombre from parametros" w418] -> w326
              tunnel: w315 -> [_ w415]
              tunnel: w314 -> [w412 _]
              frame False {
                n210 = local write "disponibilidad dori"(w412) -> ()
                n211 = One Button Dialog(message="Doritos Insuficientes") -> ()  [unwired: 1 in, 1 out]
              }
              frame True {
                n212 = local write "disponibilidad dori"(w415) -> ()
                n213 = Number To Decimal String(number=w417) -> (decimal integer string=w420:string)  [unwired: 1 in]
                n214 = Concatenate Strings("update parametros SET disponibilidad='", w420, " ' where nombre='doritos';" ("string")) -> (w418:string)
              }
            }
            n215 = case shown="False" w339 {
              tunnel: w316 -> [_ w429]
              tunnel: ["select nombre from parametros" w425] -> w328
              tunnel: w317 -> [w422 _]
              tunnel: w316 -> [_ w424]
              frame False {
                n216 = local write "disponibilidad chee"(w422) -> ()
                n217 = One Button Dialog(message="Chettos Insuficientes") -> ()  [unwired: 1 in, 1 out]
              }
              frame True {
                n218 = local write "disponibilidad chee"(w424) -> ()
                n219 = Number To Decimal String(number=w429) -> (decimal integer string=w427:string)  [unwired: 1 in]
                n220 = Concatenate Strings("update parametros SET disponibilidad='", w427, " ' where nombre='chettos';" ("string")) -> (w425:string)
              }
            }
            n221 = case shown="False" w341 {
              tunnel: w332 -> [_ w437]
              tunnel: ["select nombre from parametros" w433] -> w329
              tunnel: w318 -> [w430 _]
              frame False {
                n222 = local write "disponibilidad gans"(w430) -> ()
                n223 = One Button Dialog(message="Gansitos Insuficientes") -> ()  [unwired: 1 in, 1 out]
              }
              frame True {
                n224 = Number To Decimal String(number=w437) -> (decimal integer string=w435:string)  [unwired: 1 in]
                n225 = Concatenate Strings("update parametros SET disponibilidad='", w435, "' where nombre='gansito';" ("string")) -> (w433:string)
              }
            }
            n226 = case shown="False" w343 {
              tunnel: w320 -> [_ w446]
              tunnel: ["select nombre from parametros" w442] -> w330
              tunnel: w320 -> [_ w441]
              tunnel: w319 -> [w438 _]
              frame False {
                n227 = local write "Disponibilidad chi"(w438) -> ()
                n228 = One Button Dialog(message="Chips Insuficientes") -> ()  [unwired: 1 in, 1 out]
              }
              frame True {
                n229 = local write "Disponibilidad chi"(w441) -> ()
                n230 = Number To Decimal String(number=w446) -> (decimal integer string=w444:string)  [unwired: 1 in]
                n231 = Concatenate Strings("update parametros SET disponibilidad='", w444, "' where nombre='chips';" ("string")) -> (w442:string)
              }
            }
            n232 = case shown="False" w346 {
              tunnel: w322 -> [_ w453]
              tunnel: ["select nombre from parametros" w454] -> w331
              tunnel: w322 -> [_ w450]
              tunnel: w321 -> [w447 _]
              frame False {
                n233 = local write "disponibilidad tak"(w447) -> ()
                n234 = One Button Dialog(message="Takis Insuficientes") -> ()  [unwired: 1 in, 1 out]
              }
              frame True {
                n235 = local write "disponibilidad tak"(w450) -> ()
                n236 = Number To Decimal String(number=w453) -> (decimal integer string=w452:string)  [unwired: 1 in]
                n237 = Concatenate Strings("update parametros SET disponibilidad='", w452, "' where nombre='takis';" ("string")) -> (w454:string)
              }
            }
            n238 = local read "UDL"() -> (w372:path)
            n239 = call-poly <vilib>:"DB Tools Open Connection.vi"("connection information"=w372) -> ("error out"=w373:errorcluster, "connection reference"=w352:T5)  [unwired: 7 in]
            n240 = call-poly <vilib>:"DB Tools Open Connection.vi"("connection information"=w372) -> ("error out"=w378:errorcluster, "connection reference"=w356:T5)  [unwired: 7 in]
            n241 = call-poly <vilib>:"DB Tools Open Connection.vi"("connection information"=w372) -> ("error out"=w383:errorcluster, "connection reference"=w360:T5)  [unwired: 7 in]
            n242 = call-poly <vilib>:"DB Tools Open Connection.vi"("connection information"=w372) -> ("error out"=w388:errorcluster, "connection reference"=w364:T5)  [unwired: 7 in]
            n243 = call-poly <vilib>:"DB Tools Open Connection.vi"("connection information"=w372) -> ("error out"=w393:errorcluster, "connection reference"=w367:T5)  [unwired: 7 in]
            n244 = call-poly <vilib>:"DB Tools Open Connection.vi"("connection information"=w372) -> ("error out"=w398:errorcluster, "connection reference"=w371:T5)  [unwired: 7 in]
            n245 = call-poly <vilib>:"DB Tools Execute Query.vi"("error in (no error)"=w373, "SQL query"=w323, "connection reference"=w352) -> ("error out"=w377:errorcluster, "recordset reference"=w351:T6)  [unwired: 5 in]
            n246 = call-poly <vilib>:"DB Tools Execute Query.vi"("error in (no error)"=w378, "SQL query"=w326, "connection reference"=w356) -> ("error out"=w382:errorcluster, "recordset reference"=w355:T6)  [unwired: 5 in]
            n247 = call-poly <vilib>:"DB Tools Execute Query.vi"("error in (no error)"=w383, "SQL query"=w328, "connection reference"=w360) -> ("error out"=w387:errorcluster, "recordset reference"=w359:T6)  [unwired: 5 in]
            n248 = call-poly <vilib>:"DB Tools Execute Query.vi"("error in (no error)"=w388, "SQL query"=w329, "connection reference"=w364) -> ("error out"=w392:errorcluster, "recordset reference"=w363:T6)  [unwired: 5 in]
            n249 = call-poly <vilib>:"DB Tools Execute Query.vi"("error in (no error)"=w393, "SQL query"=w330, "connection reference"=w367) -> ("error out"=w397:errorcluster, "recordset reference"=w366:T6)  [unwired: 5 in]
            n250 = call-poly <vilib>:"DB Tools Execute Query.vi"("error in (no error)"=w398, "SQL query"=w331, "connection reference"=w371) -> ("error out"=w402:errorcluster, "recordset reference"=w370:T6)  [unwired: 5 in]
            n251 = call-poly <vilib>:"DB Tools Fetch Recordset Data.vi"("error in (no error)"=w377, "recordset reference"=w351) -> ("error out"=w374:errorcluster, "recordset reference out"=w350:T6)  [unwired: 3 in, 1 out]
            n252 = call-poly <vilib>:"DB Tools Fetch Recordset Data.vi"("error in (no error)"=w382, "recordset reference"=w355) -> ("error out"=w379:errorcluster, "recordset reference out"=w354:T6)  [unwired: 3 in, 1 out]
            n253 = call-poly <vilib>:"DB Tools Fetch Recordset Data.vi"("error in (no error)"=w387, "recordset reference"=w359) -> ("error out"=w384:errorcluster, "recordset reference out"=w358:T6)  [unwired: 3 in, 1 out]
            n254 = call-poly <vilib>:"DB Tools Fetch Recordset Data.vi"("error in (no error)"=w392, "recordset reference"=w363) -> ("error out"=w389:errorcluster, "recordset reference out"=w362:T6)  [unwired: 3 in, 1 out]
            n255 = call-poly <vilib>:"DB Tools Fetch Recordset Data.vi"("error in (no error)"=w397, "recordset reference"=w366) -> ("error out"=w394:errorcluster, "recordset reference out"=w365:T6)  [unwired: 3 in, 1 out]
            n256 = call-poly <vilib>:"DB Tools Fetch Recordset Data.vi"("error in (no error)"=w402, "recordset reference"=w370) -> ("error out"=w399:errorcluster, "recordset reference out"=w369:T6)  [unwired: 3 in, 1 out]
            n257 = call-poly <vilib>:"DB Tools Free Object.vi"("error in (no error)"=w374, "recordset reference"=w350) -> ("error out"=w375:errorcluster, "connection reference"=w349:T5)  [unwired: 8 in]
            n258 = call-poly <vilib>:"DB Tools Free Object.vi"("error in (no error)"=w379, "recordset reference"=w354) -> ("error out"=w380:errorcluster, "connection reference"=w353:T5)  [unwired: 8 in]
            n259 = call-poly <vilib>:"DB Tools Free Object.vi"("error in (no error)"=w384, "recordset reference"=w358) -> ("error out"=w385:errorcluster, "connection reference"=w357:T5)  [unwired: 8 in]
            n260 = call-poly <vilib>:"DB Tools Free Object.vi"("error in (no error)"=w389, "recordset reference"=w362) -> ("error out"=w390:errorcluster, "connection reference"=w361:T5)  [unwired: 8 in]
            n261 = call-poly <vilib>:"DB Tools Free Object.vi"("error in (no error)"=w394, "recordset reference"=w365) -> ("error out"=w395:errorcluster, "connection reference"=w348:T5)  [unwired: 8 in]
            n262 = call-poly <vilib>:"DB Tools Free Object.vi"("error in (no error)"=w399, "recordset reference"=w369) -> ("error out"=w400:errorcluster, "connection reference"=w368:T5)  [unwired: 8 in]
            n263 = call <vilib>:"DB Tools Close Connection.vi"("error in (no error)"=w375, "connection reference"=w349) -> ("error out"=w376:errorcluster)  [unwired: 5 in]
            n264 = call <vilib>:"DB Tools Close Connection.vi"("error in (no error)"=w380, "connection reference"=w353) -> ("error out"=w381:errorcluster)  [unwired: 5 in]
            n265 = call <vilib>:"DB Tools Close Connection.vi"("error in (no error)"=w385, "connection reference"=w357) -> ("error out"=w386:errorcluster)  [unwired: 5 in]
            n266 = call <vilib>:"DB Tools Close Connection.vi"("error in (no error)"=w390, "connection reference"=w361) -> ("error out"=w391:errorcluster)  [unwired: 5 in]
            n267 = call <vilib>:"DB Tools Close Connection.vi"("error in (no error)"=w395, "connection reference"=w348) -> ("error out"=w396:errorcluster)  [unwired: 5 in]
            n268 = call <vilib>:"DB Tools Close Connection.vi"("error in (no error)"=w400, "connection reference"=w368) -> ("error out"=w401:errorcluster)  [unwired: 5 in]
            n269 = call <vilib>:"Simple Error Handler.vi"("error in (no error)"=w376) -> ()  [unwired: 4 in, 5 out]
            n270 = call <vilib>:"Simple Error Handler.vi"("error in (no error)"=w381) -> ()  [unwired: 4 in, 5 out]
            n271 = call <vilib>:"Simple Error Handler.vi"("error in (no error)"=w386) -> ()  [unwired: 4 in, 5 out]
            n272 = call <vilib>:"Simple Error Handler.vi"("error in (no error)"=w391) -> ()  [unwired: 4 in, 5 out]
            n273 = call <vilib>:"Simple Error Handler.vi"("error in (no error)"=w396) -> ()  [unwired: 4 in, 5 out]
            n274 = call <vilib>:"Simple Error Handler.vi"("error in (no error)"=w401) -> ()  [unwired: 4 in, 5 out]
          }
        }
      }
      event "cheetos": Value Change {
        n275 = event-data() -> ()  [unwired: 1 in, 6 out]
        n276 = local read "UDL"() -> (w464:path)
        n277 = Concatenate Strings("SELECT precio FROM parametros where nombre='cheetos';") -> (w460:string)
        n278 = call-poly <vilib>:"DB Tools Open Connection.vi"("connection information"=w464) -> ("error out"=w470:errorcluster, "connection reference"=w469:T5)  [unwired: 7 in]
        n279 = local read "SaldoAux"() -> (w463:dbl)
        n280 = Decimal String To Number(string=w460) -> (number=w465:i32)  [unwired: 2 in, 1 out]
        n281 = call-poly <vilib>:"DB Tools Execute Query.vi"("error in (no error)"=w470, "SQL query"=w460, "connection reference"=w469) -> ("error out"=w474:errorcluster, "recordset reference"=w468:T6)  [unwired: 5 in]
        n282 = Greater?(x=w463, y=w465) -> (0:w462:bool)
        n283 = call-poly <vilib>:"DB Tools Fetch Recordset Data.vi"("error in (no error)"=w474, "recordset reference"=w468) -> ("error out"=w471:errorcluster, "recordset reference out"=w467:T6)  [unwired: 3 in, 1 out]
        n284 = call-poly <vilib>:"DB Tools Free Object.vi"("error in (no error)"=w471, "recordset reference"=w467) -> ("error out"=w472:errorcluster, "connection reference"=w466:T5)  [unwired: 8 in]
        n285 = call <vilib>:"DB Tools Close Connection.vi"("error in (no error)"=w472, "connection reference"=w466) -> ("error out"=w473:errorcluster)  [unwired: 5 in]
        n286 = case shown="True" w462 {
          tunnel: w464 -> [_ w484]
          tunnel: [_ w483] -> w459
          tunnel: [_ w482] -> w458
          tunnel: w457 -> [_ w480]
          tunnel: w456 -> [_ w479]
          frame False {
            n287 = One Button Dialog(message="Saldo Insuficiente") -> ()  [unwired: 1 in, 1 out]
          }
          frame True {
            n288 = local read "cheetos"() -> (w481:bool)
            n289 = case shown="True" w481 {
              tunnel: w480 -> [_ w506]
              tunnel: [_ w505] -> w483
              tunnel: w479 -> [_ w503]
              tunnel: [_ w502] -> w482
              frame False {
              }
              frame True {
                n290 = while {
                  tunnel: w506 -> [w516]
                  tunnel: [w517] -> w505
                  shift-right: [w510] -> _
                  shift-left: bool[] [TRUE, FALSE, FALSE, TRUE] ("data") -> [w514]
                  tunnel: w503 -> [w509]
                  tunnel: [w508] -> w502
                  i -> [w511]
                  stop <- w512 stop-if-true
                  n291 = call-poly <vilib>:"DAQmx Write.vi"("task/channels in"=w516, "data"=w514, "error in"=w509) -> ("task out"=w517:refnum<k21>, "error out"=w508:errorcluster)  [unwired: 10 in, 1 out]
                  n292 = Rotate 1D Array(1:w514, 2:1 ("n")) -> (0:w510:bool[])
                  n293 = Equal?(x=w511, y=3000) -> (x = y?=w512:bool)
                  n294 = Wait Until Next ms Multiple(millisecond multiple=u32 3) -> ()  [unwired: 1 out]
                  "Numeric 3" <- w511
                }
              }
            }
            n295 = Decrement(x="disponibilidad chee") -> (x-1=w476:dbl)
            n296 = Greater Than 0?(x=w476) -> (x > 0?=w478:bool)
            n297 = local write "disponibilidad chee"(w476) -> ()
            n298 = Less Than 0?(x=w476) -> (x < 0?=w494:bool)
            n299 = Number To Decimal String(number=w476) -> (decimal integer string=w485:string)  [unwired: 1 in]
            n300 = case shown="True" w478 {
              tunnel: [u16 0 ("crujos") u16 1 ("crujos")] -> w477
              frame False {
              }
              frame True {
              }
            }
            "cheetines" <- w477
            n301 = case shown="True" w494 {
              frame False {
              }
              frame True {
                n302 = local write "disponibilidad chee"(0.0 ("TAKIS")) -> ()
              }
            }
            n303 = Concatenate Strings("UPDATE parametros SET disponibilidad='", w485, "' where nombre='chettos';") -> (w493:string)
            n304 = call-poly <vilib>:"DB Tools Open Connection.vi"("connection information"=w484) -> ("error out"=w487:errorcluster, "connection reference"=w498:T5)  [unwired: 7 in]
            n305 = call-poly <vilib>:"DB Tools Execute Query.vi"("error in (no error)"=w487, "SQL query"=w493, "connection reference"=w498) -> ("error out"=w488:errorcluster, "recordset reference"=w499:T6)  [unwired: 5 in]
            n306 = call-poly <vilib>:"DB Tools Fetch Recordset Data.vi"("error in (no error)"=w488, "recordset reference"=w499) -> ("error out"=w489:errorcluster, "recordset reference out"=w497:T6)  [unwired: 3 in, 1 out]
            n307 = call-poly <vilib>:"DB Tools Free Object.vi"("error in (no error)"=w489, "recordset reference"=w497) -> ("error out"=w490:errorcluster, "connection reference"=w496:T5)  [unwired: 8 in]
            n308 = call <vilib>:"DB Tools Close Connection.vi"("error in (no error)"=w490, "connection reference"=w496) -> ("error out"=w491:errorcluster)  [unwired: 5 in]
            n309 = call <vilib>:"Simple Error Handler.vi"("error in (no error)"=w491) -> ()  [unwired: 4 in, 5 out]
          }
        }
        n310 = call <vilib>:"Simple Error Handler.vi"("error in (no error)"=w473) -> ()  [unwired: 4 in, 5 out]
      }
      event "takis1", "gansito1", "doritos1", "crujitos1", "chettos1": Value Change {
        n311 = event-data() -> ()  [unwired: 1 in, 6 out]
        n312 = Greater Than 0?(x="gansito1") -> (x > 0?=w532:bool)
        n313 = Greater Than 0?(x="chips1") -> (x > 0?=w534:bool)
        n314 = Greater Than 0?(x="doritos1") -> (x > 0?=w528:bool)
        n315 = Greater Than 0?(x="takis1") -> (x > 0?=w535:bool)
        n316 = Greater Than 0?(x="chettos1") -> (x > 0?=w530:bool)
        n317 = Multiply(x="takis1", y=19.0) -> (x*y=w549:dbl)
        n318 = Multiply(x="chips1", y=24.0) -> (x*y=w548:dbl)
        n319 = Multiply(x="gansito1", y=22.0) -> (x*y=w547:dbl)
        n320 = Multiply(x=15.0, y="chettos1") -> (x*y=w546:dbl)
        n321 = Multiply(x="doritos1", y=19.0) -> (x*y=w545:dbl)
        n322 = Multiply(x="crujitos1", y=17.0) -> (x*y=w544:dbl)
        n323 = Greater Than 0?(x="crujitos1") -> (x > 0?=w526:bool)
        n324 = case shown="False" w532 {
          tunnel: [u16 0 ("Ring") u16 1 ("Ring")] -> w522
          frame False {
          }
          frame True {
          }
        }
        "Gansito 2" <- w522
        n325 = case shown="True" w534 {
          tunnel: [u16 0 ("Ring") u16 1 ("Ring")] -> w523
          frame False {
          }
          frame True {
          }
        }
        "Chips 2" <- w523
        n326 = case shown="False" w526 {
          tunnel: [u16 0 ("Ring") u16 1 ("Ring")] -> w519
          frame False {
          }
          frame True {
          }
        }
        "crujos 2" <- w519
        n327 = case shown="False" w528 {
          tunnel: [u16 0 ("Ring") u16 1 ("Ring")] -> w520
          frame False {
          }
          frame True {
          }
        }
        "doros 2" <- w520
        n328 = case shown="False" w535 {
          tunnel: [u16 0 ("Ring") u16 1 ("Ring")] -> w524
          frame False {
          }
          frame True {
          }
        }
        "Takis 2" <- w524
        n329 = case shown="False" w530 {
          tunnel: [u16 0 ("Ring") u16 1 ("Ring")] -> w521
          frame False {
          }
          frame True {
          }
        }
        "cheetines 2" <- w521
        n330 = Compound Arithmetic op=ADD(w549, w548, w547, w546, w545, w544) -> (→"Total Carrito":dbl)
      }
      event "doritos": Value Change {
        n331 = event-data() -> ()  [unwired: 1 in, 6 out]
        n332 = local read "UDL"() -> (w565:path)
        n333 = Concatenate Strings("Select precio from parametros where nombre='doritos';") -> (w562:string)
        n334 = call-poly <vilib>:"DB Tools Open Connection.vi"("connection information"=w565) -> ("error out"=w572:errorcluster, "connection reference"=w571:T5)  [unwired: 7 in]
        n335 = local read "SaldoAux"() -> (w566:dbl)
        n336 = Decimal String To Number(string=w562) -> (number=w567:i32)  [unwired: 2 in, 1 out]
        n337 = call-poly <vilib>:"DB Tools Execute Query.vi"("error in (no error)"=w572, "SQL query"=w562, "connection reference"=w571) -> ("error out"=w576:errorcluster, "recordset reference"=w570:T6)  [unwired: 5 in]
        n338 = Greater?(x=w566, y=w567) -> (0:w564:bool)
        n339 = call-poly <vilib>:"DB Tools Fetch Recordset Data.vi"("error in (no error)"=w576, "recordset reference"=w570) -> ("error out"=w573:errorcluster, "recordset reference out"=w569:T6)  [unwired: 3 in, 1 out]
        n340 = call-poly <vilib>:"DB Tools Free Object.vi"("error in (no error)"=w573, "recordset reference"=w569) -> ("error out"=w574:errorcluster, "connection reference"=w568:T5)  [unwired: 8 in]
        n341 = case shown="True" w564 {
          tunnel: w565 -> [_ w581]
          frame False {
            n342 = One Button Dialog(message="Saldo Insuficiente") -> ()  [unwired: 1 in, 1 out]
          }
          frame True {
            n343 = Decrement(x="disponibilidad dori") -> (x-1=w578:dbl)
            n344 = Greater Than 0?(x=w578) -> (x > 0?=w579:bool)
            n345 = case shown="True" w579 {
              tunnel: [u16 0 ("doros") u16 1 ("doros")] -> w580
              frame False {
              }
              frame True {
              }
            }
            "doros" <- w580
            n346 = Less Than 0?(x=w578) -> (x < 0?=w591:bool)
            n347 = Number To Decimal String(number=w578) -> (decimal integer string=w583:string)  [unwired: 1 in]
            n348 = local write "disponibilidad dori"(w578) -> ()
            n349 = case shown="True" w591 {
              frame False {
              }
              frame True {
                n350 = local write "disponibilidad dori"(0.0 ("TAKIS")) -> ()
              }
            }
            n351 = Concatenate Strings("UPDATE parametros SET disponibilidad='", w583, "' where nombre='doritos';") -> (w582:string)
            n352 = call-poly <vilib>:"DB Tools Open Connection.vi"("connection information"=w581) -> ("error out"=w585:errorcluster, "connection reference"=w595:T5)  [unwired: 7 in]
            n353 = call-poly <vilib>:"DB Tools Execute Query.vi"("error in (no error)"=w585, "SQL query"=w582, "connection reference"=w595) -> ("error out"=w586:errorcluster, "recordset reference"=w596:T6)  [unwired: 5 in]
            n354 = call-poly <vilib>:"DB Tools Fetch Recordset Data.vi"("error in (no error)"=w586, "recordset reference"=w596) -> ("error out"=w587:errorcluster, "recordset reference out"=w594:T6)  [unwired: 3 in, 1 out]
            n355 = call-poly <vilib>:"DB Tools Free Object.vi"("error in (no error)"=w587, "recordset reference"=w594) -> ("error out"=w588:errorcluster, "connection reference"=w593:T5)  [unwired: 8 in]
            n356 = call <vilib>:"DB Tools Close Connection.vi"("error in (no error)"=w588, "connection reference"=w593) -> ("error out"=w589:errorcluster)  [unwired: 5 in]
            n357 = call <vilib>:"Simple Error Handler.vi"("error in (no error)"=w589) -> ()  [unwired: 4 in, 5 out]
          }
        }
        n358 = call <vilib>:"DB Tools Close Connection.vi"("error in (no error)"=w574, "connection reference"=w568) -> ("error out"=w575:errorcluster)  [unwired: 5 in]
        n359 = call <vilib>:"Simple Error Handler.vi"("error in (no error)"=w575) -> ()  [unwired: 4 in, 5 out]
      }
      event "crujitos": Value Change {
        n360 = event-data() -> ()  [unwired: 1 in, 6 out]
        n361 = local read "UDL"() -> (w603:path)
        n362 = Concatenate Strings("Select precio from parametros where nombre='crujitos';") -> (w600:string)
        n363 = call-poly <vilib>:"DB Tools Open Connection.vi"("connection information"=w603) -> ("error out"=w610:errorcluster, "connection reference"=w609:T5)  [unwired: 7 in]
        n364 = local read "SaldoAux"() -> (w604:dbl)
        n365 = Decimal String To Number(string=w600) -> (number=w605:i32)  [unwired: 2 in, 1 out]
        n366 = call-poly <vilib>:"DB Tools Execute Query.vi"("error in (no error)"=w610, "SQL query"=w600, "connection reference"=w609) -> ("error out"=w614:errorcluster, "recordset reference"=w608:T6)  [unwired: 5 in]
        n367 = Greater?(x=w604, y=w605) -> (0:w602:bool)
        n368 = call-poly <vilib>:"DB Tools Fetch Recordset Data.vi"("error in (no error)"=w614, "recordset reference"=w608) -> ("error out"=w611:errorcluster, "recordset reference out"=w607:T6)  [unwired: 3 in, 1 out]
        n369 = call-poly <vilib>:"DB Tools Free Object.vi"("error in (no error)"=w611, "recordset reference"=w607) -> ("error out"=w612:errorcluster, "connection reference"=w606:T5)  [unwired: 8 in]
        n370 = case shown="True" w602 {
          tunnel: w603 -> [_ w619]
          frame False {
            n371 = One Button Dialog(message="Saldo Insuficiente") -> ()  [unwired: 1 in, 1 out]
          }
          frame True {
            n372 = Decrement(x="disponibilidad cruji") -> (x-1=w616:dbl)
            n373 = Greater Than 0?(x=w616) -> (x > 0?=w617:bool)
            n374 = case shown="True" w617 {
              tunnel: [u16 0 ("crujos") u16 1 ("crujos")] -> w618
              frame False {
              }
              frame True {
              }
            }
            "crujos" <- w618
            n375 = local write "disponibilidad cruji"(w616) -> ()
            n376 = Less Than 0?(x=w616) -> (x < 0?=w629:bool)
            n377 = Number To Decimal String(number=w616) -> (decimal integer string=w620:string)  [unwired: 1 in]
            n378 = case shown="True" w629 {
              frame False {
              }
              frame True {
                n379 = local write "disponibilidad cruji"(0.0 ("TAKIS")) -> ()
              }
            }
            n380 = Concatenate Strings("UPDATE parametros SET disponibilidad='", w620, "' where nombre='crujitos';") -> (w628:string)
            n381 = call-poly <vilib>:"DB Tools Open Connection.vi"("connection information"=w619) -> ("error out"=w622:errorcluster, "connection reference"=w633:T5)  [unwired: 7 in]
            n382 = call-poly <vilib>:"DB Tools Execute Query.vi"("error in (no error)"=w622, "SQL query"=w628, "connection reference"=w633) -> ("error out"=w623:errorcluster, "recordset reference"=w634:T6)  [unwired: 5 in]
            n383 = call-poly <vilib>:"DB Tools Fetch Recordset Data.vi"("error in (no error)"=w623, "recordset reference"=w634) -> ("error out"=w624:errorcluster, "recordset reference out"=w632:T6)  [unwired: 3 in, 1 out]
            n384 = call-poly <vilib>:"DB Tools Free Object.vi"("error in (no error)"=w624, "recordset reference"=w632) -> ("error out"=w625:errorcluster, "connection reference"=w631:T5)  [unwired: 8 in]
            n385 = call <vilib>:"DB Tools Close Connection.vi"("error in (no error)"=w625, "connection reference"=w631) -> ("error out"=w626:errorcluster)  [unwired: 5 in]
            n386 = call <vilib>:"Simple Error Handler.vi"("error in (no error)"=w626) -> ()  [unwired: 4 in, 5 out]
          }
        }
        n387 = call <vilib>:"DB Tools Close Connection.vi"("error in (no error)"=w612, "connection reference"=w606) -> ("error out"=w613:errorcluster)  [unwired: 5 in]
        n388 = call <vilib>:"Simple Error Handler.vi"("error in (no error)"=w613) -> ()  [unwired: 4 in, 5 out]
      }
    }
  }
  n389 = call <vilib>:"IMAQdx Close Camera.vi"("error in"=w14, "Session In"=w16) -> ("error out"=w26:errorcluster)  [unwired: 9 in]
  n390 = call "Imaq Dispose"("Image"=w13, "error in (no error)"=w26) -> ()  [unwired: 4 in, 1 out]
  n391 = call <vilib>:"DAQmx Clear Task.vi"("task in"=w24, "error in"=w23) -> ("error out"=w25:errorcluster)  [unwired: 13 in]
  n392 = call <vilib>:"DAQmx Clear Task.vi"("task in"=w2, "error in"=w1) -> ("error out"=w3:errorcluster)  [unwired: 13 in]
  n393 = call <vilib>:"DAQmx Clear Task.vi"("task in"=w11, "error in"=w9) -> ("error out"=w10:errorcluster)  [unwired: 13 in]
  n394 = call <vilib>:"Simple Error Handler.vi"("error in (no error)"=w25) -> ()  [unwired: 4 in, 5 out]
  n395 = call <vilib>:"Simple Error Handler.vi"("error in (no error)"=w3) -> ()  [unwired: 4 in, 5 out]
  n396 = call <vilib>:"Simple Error Handler.vi"("error in (no error)"=w10) -> ()  [unwired: 4 in, 5 out]
